vi "CII.vi"(0 "Wheel":dbl, 1 "Throttle":dbl) -> (7 "RightDrive":dbl, 8 "LeftDrive":dbl)   [LabVIEW 2014]
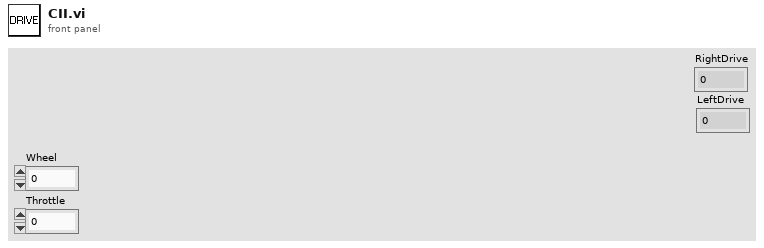
[diagram p1: front panel]
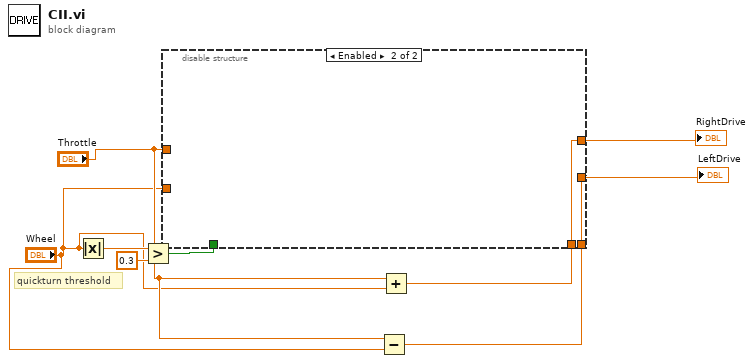
[diagram p0: block diagram]
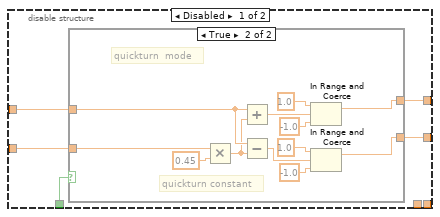
[diagram p2: hidden frame]
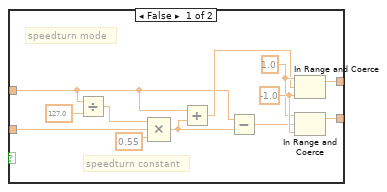
[diagram p3: hidden frame]
diagram:
  # "quickturn threshold"
  n1 = Absolute Value(x="Wheel") -> (abs(x)=w9:dbl)
  n2 = Greater?(x=w9, y=0.3) -> (0:w8:bool)
  n3 = Subtract(x="Throttle", y="Wheel") -> (x-y=w1:dbl)
  n4 = Add(x="Throttle", y="Wheel") -> (x+y=w2:dbl)
  n5 = disable-structure shown="Enabled" {
    disable-tunnel: w8 -> [w14 _]
    disable-tunnel: [w13 w40] -> w6
    disable-tunnel: [w12 w39] -> w5
    disable-tunnel: "Throttle" -> [w11 _]
    disable-tunnel: "Wheel" -> [w10 _]
    disable-tunnel: w2 -> [_ w40]
    disable-tunnel: w1 -> [_ w39]
    frame Disabled {
      n6 = case shown="True" w14 {
        tunnel: w11 -> [w15 w36]
        tunnel: w10 -> [w18 w38]
        tunnel: [w22 w29] -> w13
        tunnel: [w21 w32] -> w12
        frame False {
          w20 = -1.0 ("upper limit")
          w19 = 1.0 ("milliseconds to wait")
          # "speedturn constant"
          # "speedturn mode"
          n7 = Divide(x=w15, y=127.0) -> (x/y=w25:dbl)
          n8 = Compound Arithmetic op=MULTIPLY(w25, w18, 0.55) -> (w23:dbl)
          n9 = Add(x=w15, y=w23) -> (x+y=w16:dbl)
          n10 = Subtract(x=w15, y=w23) -> (x-y=w17:dbl)
          n11 = In Range and Coerce(upper limit=w19, x=w16, lower limit=w20) -> (coerced(x)=w22:dbl)  [unwired: 1 out]
          n12 = In Range and Coerce(upper limit=w19, x=w17, lower limit=w20) -> (coerced(x)=w21:dbl)  [unwired: 1 out]
        }
        frame True {
          # "quickturn constant"
          # "quickturn  mode"
          n13 = Multiply(x=w38, y=0.45) -> (x*y=w35:dbl)
          n14 = Add(x=w36, y=w35) -> (x+y=w28:dbl)
          n15 = Subtract(x=w36, y=w35) -> (x-y=w27:dbl)
          n16 = In Range and Coerce(upper limit=1.0, x=w28, lower limit=-1.0) -> (coerced(x)=w29:dbl)  [unwired: 1 out]
          n17 = In Range and Coerce(upper limit=1.0, x=w27, lower limit=-1.0 ("upper limit")) -> (coerced(x)=w32:dbl)  [unwired: 1 out]
        }
      }
    }
    frame Enabled {
    }
  }
  "RightDrive" <- w6
  "LeftDrive" <- w5
